vi "Resample (constant to variable, multi-channel).vi"(5 "anti-aliasing?":bool=TRUE, 6 "FIR filter specifications":T1={"alias rejection (dB)"=120.0, "normalized bandwidth"=0.4536} {"normalized bandwidth" format="%.4f"; "alias rejection (dB)" format="%.2f"}, 7 "reset?":bool, 8 "error in (no error)":errorcluster, 10 "Time":dbl[](array[numeric]), 11 "X":dbl[][](array[numeric])) -> (0 "error out":errorcluster, 2 "Time Stamps":dbl[](array[numeric]) format="%#.6g", 3 "Y":dbl[][](array[numeric]))   [LabVIEW 2014, in "NI_AALPro.lvlib"]
doc: "Resamples input signal <B>X</B> according to <B>Time</B> using an FIR filter implementation. Wire data to the <B>X</B> input to determine the polymorphic instance to use or manually select the instance."
uses:
  NI_AALPro.lvlib
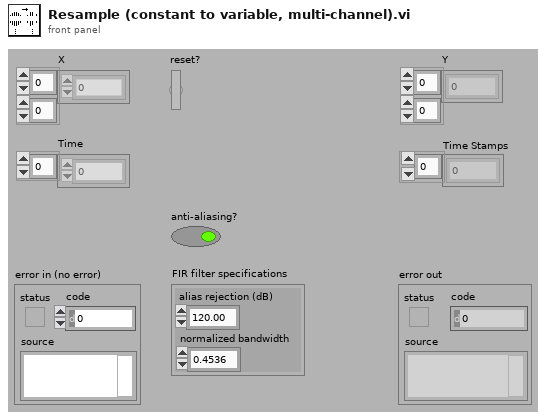
[diagram p1: front panel]
types:
  T1 = cluster{"alias rejection (dB)":dbl, "normalized bandwidth":dbl}
  T2 = cluster{"status":bool, "time not in ascending order":i32, "source":string}
  T3 = cluster{"timing jitter":enum32{"Interpolation", "Rounding"}, "anti-aliasing?":bool, "filter prototype":cluster{"coefficients":dbl[], "factor":i32}}
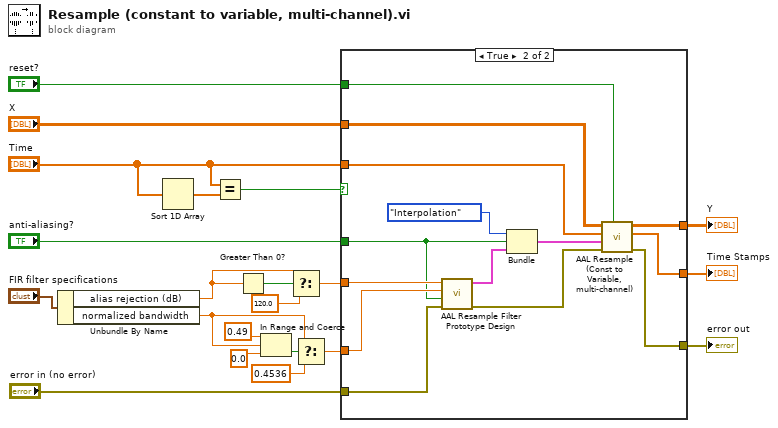
[diagram p0: block diagram]
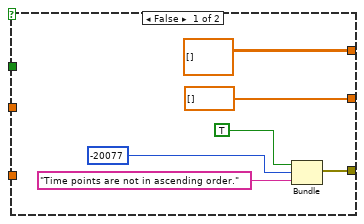
[diagram p2: hidden frame]
diagram:
  n1 = Unbundle By Name("FIR filter specifications") -> ("alias rejection (dB)"=w4:dbl, "normalized bandwidth"=w5:dbl)
  n2 = Sort 1D Array(array="Time") -> (sorted array=w14:dbl[])
  n3 = Equal?(x="Time", y=w14) -> (x = y?=w12:bool)
  n4 = Greater Than 0?(x=w4) -> (x > 0?=w3:bool)
  n5 = In Range and Coerce(upper limit=0.49, x=w5, lower limit=0.0 ("upper limit")) -> (In Range?=w7:bool)  [unwired: 1 out]
  n6 = Select(t=w4, s=w3, f=120.0) -> (s? t:f=w2:dbl)
  n7 = Select(t=w5, s=w7, f=0.4536 ("upper limit")) -> (s? t:f=w1:dbl)
  n8 = case shown="True" w12 {
    tunnel: "anti-aliasing?" -> [_ w28]
    tunnel: [dbl[][] [] ("Y") w38] -> w20
    tunnel: [w22 w37] -> w19
    tunnel: "error in (no error)" -> [_ w36]
    tunnel: "reset?" -> [_ w35]
    tunnel: "X" -> [_ w34]
    tunnel: "Time" -> [_ w33]
    tunnel: [dbl[] [] ("time stamps") w32] -> w15
    tunnel: w2 -> [_ w30]
    tunnel: w1 -> [_ w29]
    frame False {
      n9 = Bundle("status"=TRUE, "time not in ascending order"=-20077, "source"="Time points are not in ascending order.") -> (w22:T2)  [unwired: 1 in]
    }
    frame True {
      n10 = call "AAL Resample Filter Prototype Design.vi"("error in (no error)"=w36, "alias free"=w28, "normalized bandwidth"=w29, "A stop [dB]"=w30) -> ("error out"=w41:errorcluster, "filter prototype"=w40:cluster{"coefficients":dbl[], "factor":i32})  [unwired: 5 in, 1 out]
      n11 = Bundle("timing jitter"=enum32{"Interpolation", "Rounding"}."Interpolation", "anti-aliasing?"=w28, "filter prototype"=w40) -> (w39:T3)  [unwired: 1 in]
      n12 = call "AAL Resample (Const to Variable, multi-channel).vi"("reset? (True)"=w35, "error in (no error)"=w41, "config"=w39, "time"=w33, "X"=w34) -> ("error out"=w37:errorcluster, "time stamps"=w32:dbl[], "Y"=w38:dbl[][])  [unwired: 3 in, 1 out]
    }
  }
  "error out" <- w19
  "Y" <- w20
  "Time Stamps" <- w15
